vi "EMV Flow Detector.vi"(8 "error in (no error)":errorcluster, 10 "ERD Data":T1, 11 ".NET Refnum in":refnum<k24>) -> (0 "error out":errorcluster, 2 "Flow Detect":string[][](array[string]), 3 ".NET Refnum out":refnum<k24>)   [LabVIEW 2016]
uses:
  Drivers/GEA3 Toolkit/LabVIEW GEA3 Rev2 API Toolkit LV2016/Water Heating Specific/Type Definitions/GEA3 HEWH ERD Data.ctl
  Drivers/GEA3 Toolkit/LabVIEW GEA3 Rev2 API Toolkit LV2016/Water Heating Specific/Type Definitions/GEA3 HEWH Mixing Valve.ctl
  C:/TechnologyLab/NI-2010/Drivers/GEA3 Toolkit/GEA3 DLL Source/GeaCommunication.dll
  Drivers/GEA3 Toolkit/GEA3 DLL Source/GeaCommunication.dll
panel:
  in  "Detection Slope":dbl=0.5 format="%#_13g"
  out "T6 T7 Flow Dectection":bool
  out "Slope History":dbl[](array[numeric])
  out "Current T6 Temperatures Output":dbl[](array[numeric])=[75.0, 75.0, 75.0, 75.0, 75.0, 75.0, 75.0, 75.0, 75.0, 75.0, 75.0]
  out "Slope Chart T7":dbl(graph)
  out "Current T7 Temperatures":dbl[](array[numeric])
  in  "Abnormal Input Temperature":dbl=80.0
  out "Flow Dectection":bool
  out "T7 Flow Dectection":bool
  in  "Entry":dbl=11.0
  in  "POLLING_TIME_MS":dbl=1000.0
  in  "FLOW_COUNTER_MAX":dbl=15.0
  in  "STARTING_TEMPERATURE":dbl=140.0
  in  "FLOW_COUNTER_THRESHOLD":dbl=1.0
  in  "T6_OFFSET_FROM_TARGET_INDICATING_FLOW":dbl=3.0
  in  "T7_DELTA_INDICATING_FLOW":dbl=10.0
  in  "T6_DELTA_INDICATING_FLOW":dbl=2.0
  in  "T7_DELTA_FLOW_THRESHOLD":dbl=0.5
  in  "T7 STOP-T6 FLOW -THRESHOLD":dbl=4.0
  out "T6 Flow Dectection":bool
  # "reading now == 0\nreading in the past == 10"
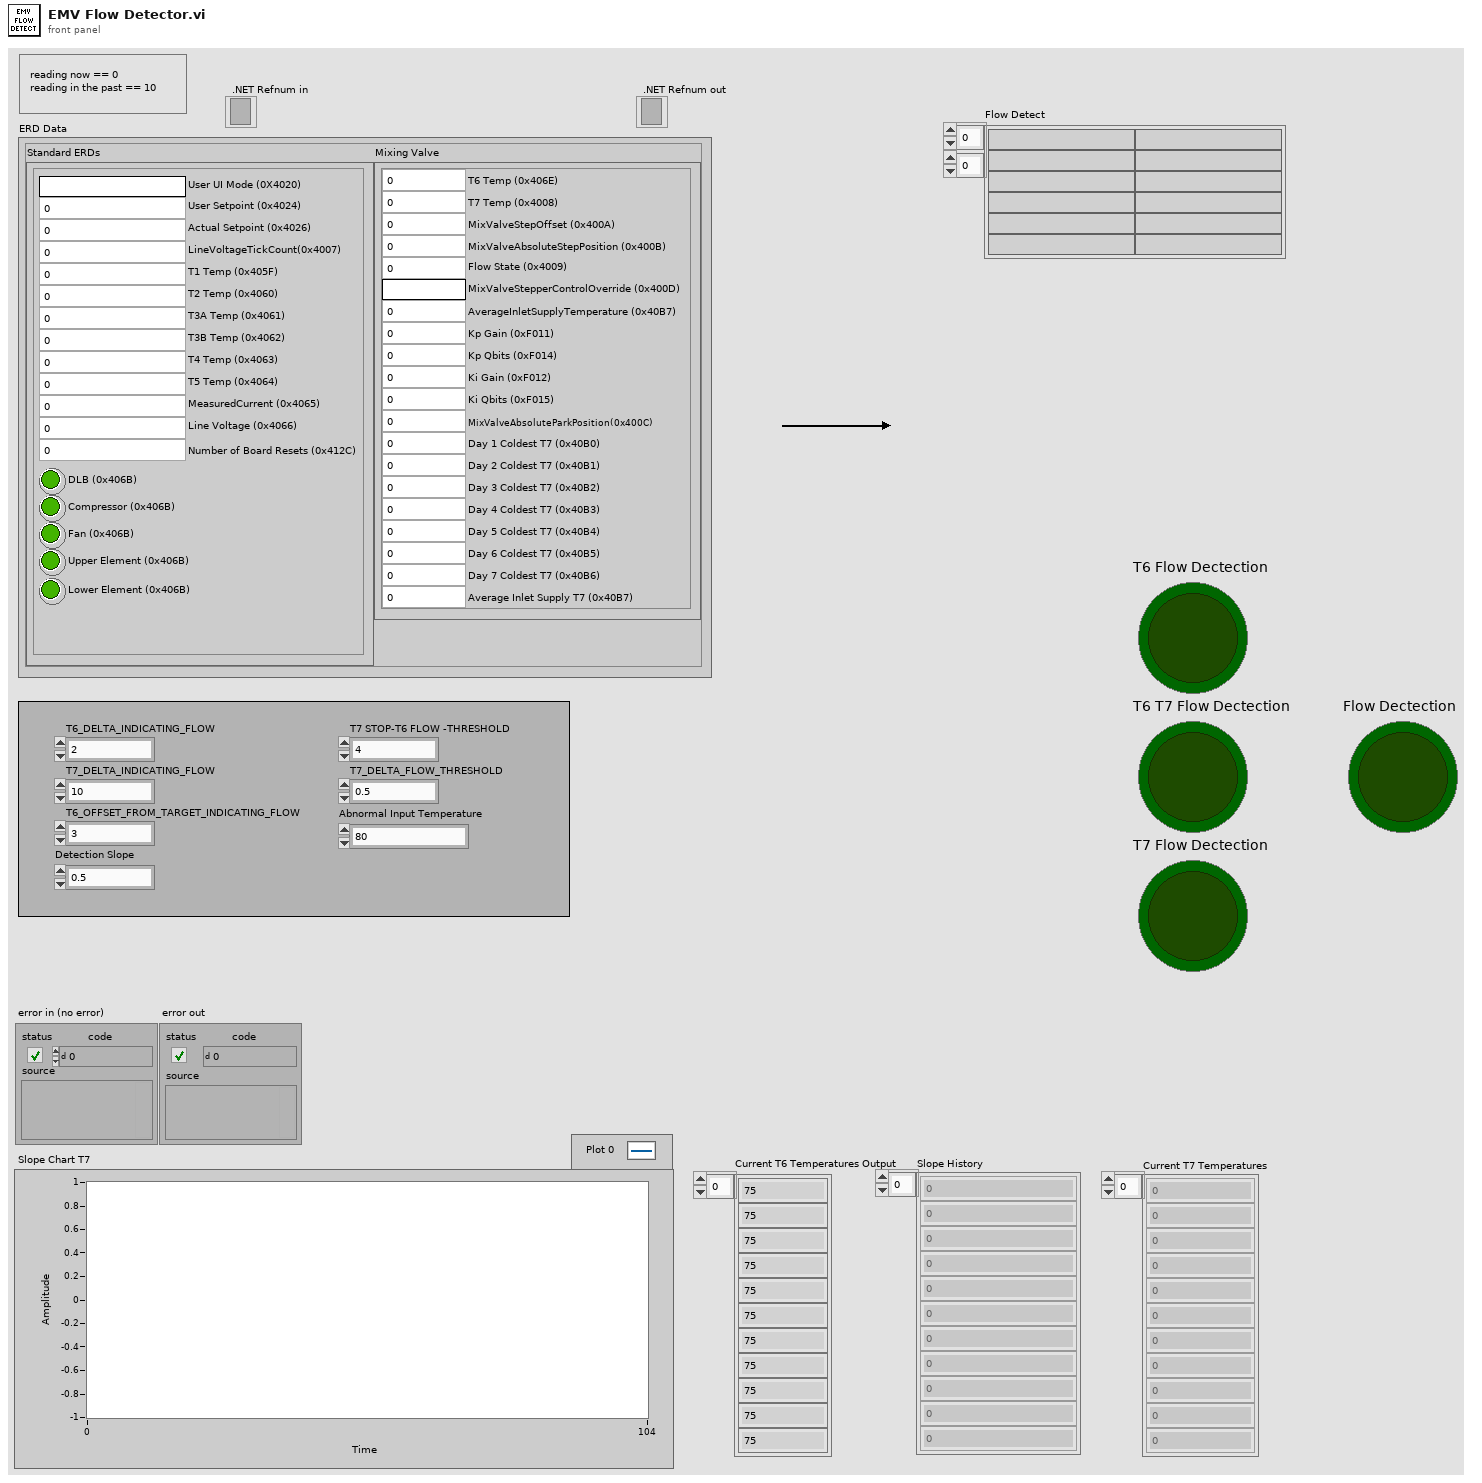
[diagram p1: front panel]
types:
  T1 = typedef "GEA3 HEWH ERD Data.ctl" = cluster{"Mixing Valve":T2, "Standard ERDs":cluster{"User UI Mode (0X4020)":string, "User Setpoint (0x4024)":u16, "Actual Setpoint (0x4026)":u16, "DLB (0x406B)":bool, "Compressor (0x406B)":bool, "Lower Element (0x406B)":bool, "Upper Element (0x406B)":bool, "Fan (0x406B)":bool, "T1 Temp (0x405F)":dbl, "T2 Temp (0x4060)":dbl, "T3A Temp (0x4061)":dbl, "T3B Temp (0x4062)":dbl, "T4 Temp (0x4063)":dbl, "T5 Temp (0x4064)":dbl, "Line Voltage (0x4066)":dbl, "MeasuredCurrent (0x4065)":dbl, "LineVoltageTickCount(0x4007)":u16, "Number of Board Resets (0x412C)":u16}}
  T2 = typedef "GEA3 HEWH Mixing Valve.ctl" = cluster{"T7 Temp (0x4008)":dbl, "MixValveStepOffset (0x400A)":i16, "MixValveAbsoluteStepPosition (0x400B)":i16, "Flow State (0x4009)":u8, "MixValveStepperControlOverride (0x400D)":string, "AverageInletSupplyTemperature (0x40B7)":dbl, "T6 Temp (0x406E)":dbl, "Kp Gain (0xF011)":u16, "Kp Qbits (0xF014)":u16, "Ki Gain (0xF012)":u16, "Ki Qbits (0xF015)":u16, "MixValveAbsoluteParkPosition(0x400C)":i16, "Day 2 Coldest T7 (0x40B1)":dbl, "Day 1 Coldest T7 (0x40B0)":dbl, "Day 4 Coldest T7 (0x40B3)":dbl, "Day 3 Coldest T7 (0x40B2)":dbl, "Day 6 Coldest T7 (0x40B5)":dbl, "Day 5 Coldest T7 (0x40B4)":dbl, "Average Inlet Supply T7 (0x40B7)":dbl, "Day 7 Coldest T7 (0x40B6)":dbl}
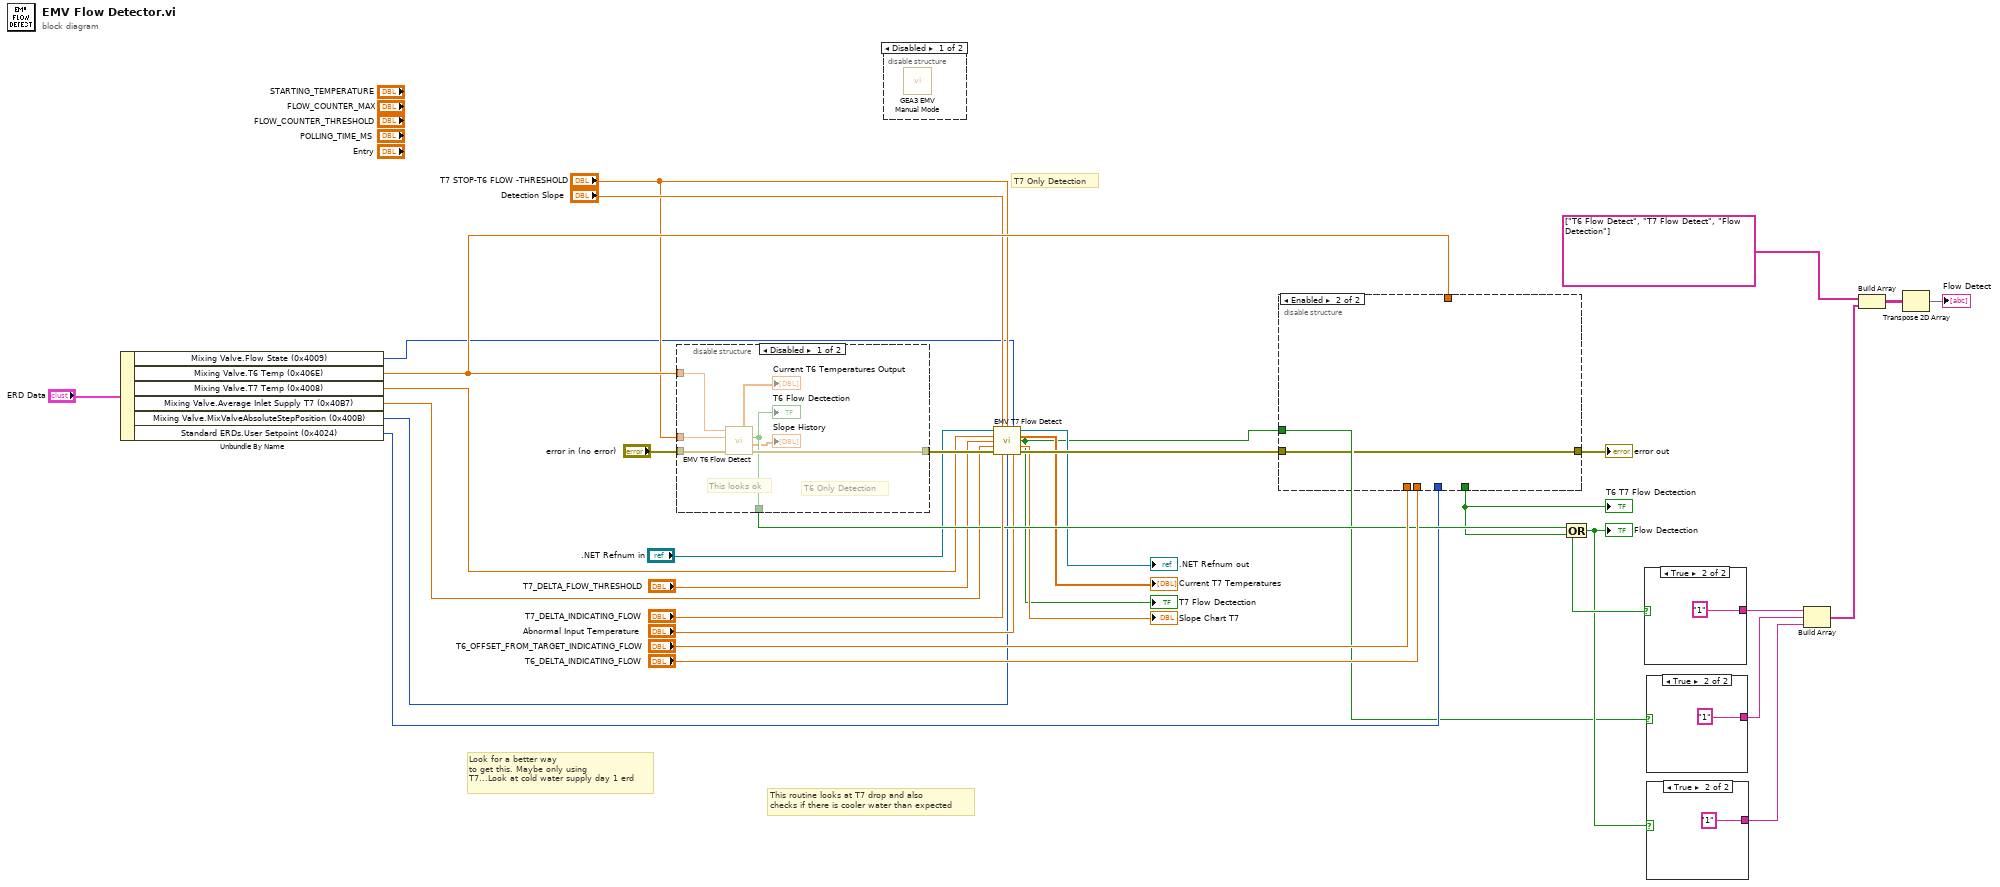
[diagram p0: block diagram]
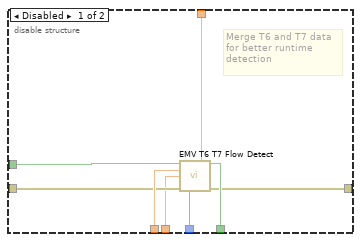
[diagram p2: hidden frame]
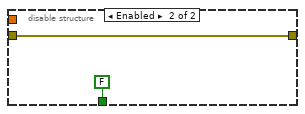
[diagram p4: hidden frame]
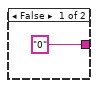
[diagram p5: hidden frame]
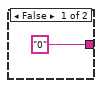
[diagram p6: hidden frame]
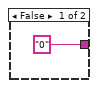
[diagram p7: hidden frame]
diagram:
  # "T7 Only Detection"
  # "Look for a better way\nto get this. Maybe only using\nT7...Look at cold water supply day 1 erd"
  # "This routine looks at T7 drop and also\nchecks if there is cooler water than expected"
  n1 = Unbundle By Name("ERD Data") -> ("Mixing Valve.Flow State (0x4009)"=w2:u8, "Mixing Valve.T6 Temp (0x406E)"=w13:dbl, "Mixing Valve.T7 Temp (0x4008)"=w5:dbl, "Mixing Valve.Average Inlet Supply T7 (0x40B7)"=w17:dbl, "Mixing Valve.MixValveAbsoluteStepPosition (0x400B)"=w8:i16, "Standard ERDs.User Setpoint (0x4024)"=w9:u16)
  n2 = disable-structure shown="Disabled" {
    disable-tunnel: "T7 STOP-T6 FLOW -THRESHOLD" -> [w40 _]
    disable-tunnel: "error in (no error)" -> [w39 w42]
    disable-tunnel: [w38 w42] -> w31
    disable-tunnel: [w36 FALSE ("Flow Dectection")] -> w26
    disable-tunnel: w13 -> [w34 _]
    frame Disabled {
      # "T6 Only Detection"
      # "This looks ok"
      n3 = call "EMV T6 Flow Detect.vi"("error in (no error)"=w39, "T6_DELTA_FLOW_THRESHOLD"=w40, "T6 Temp"=w34) -> ("error out"=w38:errorcluster, "Slope History"=→"Slope History":dbl[], "Flow Dectection"=w36:bool, "Current T6 Temperatures Output"=→"Current T6 Temperatures Output":dbl[])  [unwired: 5 in]
      "T6 Flow Dectection" <- w36
    }
    frame Enabled {
    }
  }
  n4 = disable-structure shown="Disabled" {
    frame Disabled {
      n5 = call "GEA3 EMV Manual Mode.vi"() -> ()  [unwired: 10 in, 2 out]
    }
    frame Enabled {
    }
  }
  n6 = call "EMV T7 Flow Detect.vi"(".NET Refnum in"=".NET Refnum in", "Detection Slope"="Detection Slope", "T7 STOP-T6 FLOW -THRESHOLD"="T7 STOP-T6 FLOW -THRESHOLD", "Mixing Valve.Flow State (0x4009)"=w2, "T7 Temp"=w5, "T7_DELTA_FLOW_THRESHOLD"="T7_DELTA_FLOW_THRESHOLD", "Cold Water Supply Temperature"=w17, "error in (no error)"=w31, "T7_DELTA_INDICATING_FLOW"="T7_DELTA_INDICATING_FLOW", "Mixing Valve.MixValveAbsoluteStepPosition (0x400B)"=w8, "Abnormal Input Temperature"="Abnormal Input Temperature") -> (".NET Refnum out"=→".NET Refnum out":refnum<k24>, "Current T7 Temperatures"=→"Current T7 Temperatures":dbl[], "T7 Detect?"=w1:bool, "T7 Slope Chart"=→"Slope Chart T7":dbl, "error out"=w30:errorcluster)
  "T7 Flow Dectection" <- w1
  n7 = disable-structure shown="Enabled" {
    disable-tunnel: "T6_OFFSET_FROM_TARGET_INDICATING_FLOW" -> [w50 _]
    disable-tunnel: w30 -> [w49 w51]
    disable-tunnel: "T6_DELTA_INDICATING_FLOW" -> [w48 _]
    disable-tunnel: w13 -> [w47 _]
    disable-tunnel: [w46 _] -> w12
    disable-tunnel: w9 -> [w45 _]
    disable-tunnel: [w44 w51] -> w7
    disable-tunnel: w1 -> [w43 _]
    frame Disabled {
      # "Merge T6 and T7 data\nfor better runtime \ndetection"
      n8 = call "EMV T6 T7 Flow Detect.vi"("T7 Detect?"=w43, "Mixing Valve.T6 Temp (0x406E)"=w47, "T6_OFFSET_FROM_TARGET_INDICATING_FLOW"=w50, "T6_DELTA_INDICATING_FLOW"=w48, "error in (no error)"=w49, "User Setpoint Temperature"=w45) -> ("Flow Dectection"=w46:bool, "error out"=w44:errorcluster)  [unwired: 8 in]
    }
    frame Enabled {
    }
  }
  "error out" <- w7
  "T6 T7 Flow Dectection" <- w12
  n9 = Compound Arithmetic op=OR(w26, w12) -> (w25:bool)
  "Flow Dectection" <- w25
  n10 = case shown="True" w26 {
    tunnel: ["0" "1"] -> w24
    frame False {
    }
    frame True {
    }
  }
  n11 = case shown="True" w1 {
    tunnel: ["0" "1"] -> w23
    frame False {
    }
    frame True {
    }
  }
  n12 = case shown="True" w25 {
    tunnel: ["0" "1"] -> w22
    frame False {
    }
    frame True {
    }
  }
  n13 = Build Array(w24, w23, w22) -> (w21:string[])
  n14 = Build Array(string[] ["T6 Flow Detect", "T7 Flow Detect", "Flow Detection"], w21) -> (w20:string[][])
  n15 = Transpose 2D Array(2D array=w20) -> (transposed array=→"Flow Detect":string[][])
